vi "FTW-ProjectItemManager-ReadLinkedProjectItem.vi"(0 "Project Item Manager":refnum<class "FTW-ProjectItemManager.lvclass">, 5 "Linked Project Item Tag":string, 11 "error in":errorcluster) -> (4 "Project Item Manager out":refnum<class "FTW-ProjectItemManager.lvclass">, 6 "ProjectItem":refnum<vi>, 15 "error out":errorcluster)   [LabVIEW 2012, in "FTW-ProjectItemManager.lvclass"]
uses:
  FTW-ProjectItemManager.lvclass
  FTW-ProjectItemManager.lvclass/FTW-ProjectItemManager.ctl
panel:
  # "Inputs"
  # "Outputs"
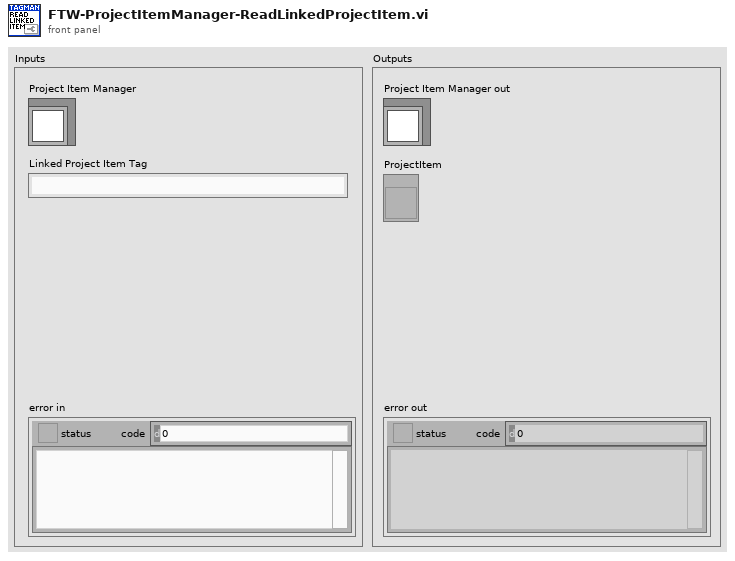
[diagram p1: front panel]
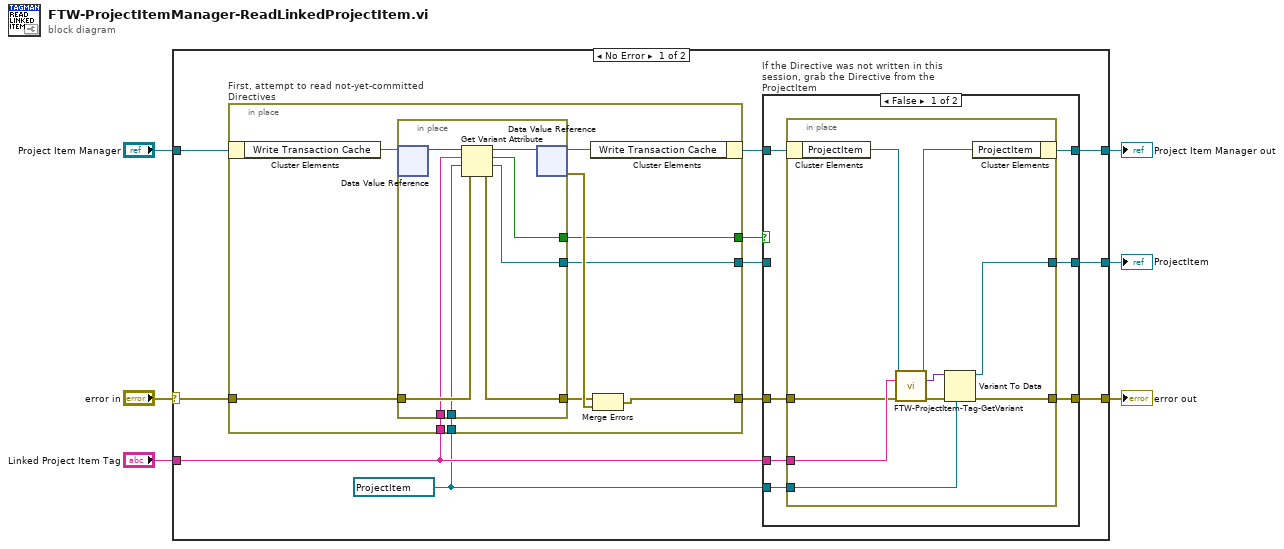
[diagram p0: block diagram]
diagram:
  n1 = case shown="No Error" "error in" {
    selector: "error in" -> [w13 w56]
    tunnel: [w7 w56] -> w6
    tunnel: [w17 w55] -> w4
    tunnel: "Project Item Manager" -> [w16 w55]
    tunnel: "Linked Project Item Tag" -> [w14 _]
    tunnel: [w8 _] -> w1
    frame No Error {
      w9 = refnum<vi> refnum ("Linked Project Item")
      n2 = in-place "First, attempt to read not-yet-committed Directives" {
        in-place-border: w13 -> [w46]
        in-place-border: [w39] -> w12
        in-place-border: w14 -> [w45]
        in-place-border: w9 -> [w44]
        in-place-border: [w38] -> w11
        in-place-border: [w37] -> w10
        n3 = in-place-cluster #1(w16) -> ("Write Transaction Cache"=w43:refnum<data-value>)
        n4 = in-place {
          in-place-border: w46 -> [w54]
          in-place-border: [w53] -> w40
          in-place-border: w45 -> [w52]
          in-place-border: w44 -> [w51]
          in-place-border: [w48] -> w38
          in-place-border: [w47] -> w37
          n5 = in-place-dvr #2(w43) -> (w50:variant)  [unwired: 1 out]
          n6 = Get Variant Attribute(Variant=w50, name=w52, default value (empty Variant)=w51, error in=w54) -> (duplicate Variant=w49:variant, found=w48:bool, value=w47:refnum<vi>, error out=w53:errorcluster)
          n7 = in-place-dvr #2(w49) -> (w42:refnum<data-value>, w41:errorcluster)
        }
        n8 = in-place-cluster #1("Write Transaction Cache"=w42) -> (w15:refnum<class "FTW-ProjectItemManager.lvclass">)
        n9 = Merge Errors(w40, w41) -> (w39:errorcluster)
      }
      n10 = case "If the Directive was not written in this\nsession, grab the Directive from the ProjectItem" shown="False" w11 {
        tunnel: [w23 w35] -> w8
        tunnel: [w18 w36] -> w17
        tunnel: [w22 w34] -> w7
        tunnel: w15 -> [w19 w36]
        tunnel: w9 -> [w24 _]
        tunnel: w14 -> [w21 _]
        tunnel: w12 -> [w20 w34]
        tunnel: w10 -> [_ w35]
        frame False {
          n11 = in-place {
            in-place-border: w24 -> [w33]
            in-place-border: [w32] -> w23
            in-place-border: [w31] -> w22
            in-place-border: w21 -> [w29]
            in-place-border: w20 -> [w28]
            n12 = in-place-cluster #3(w19) -> ("ProjectItem"=w26:refnum<vi>)
            n13 = call "FTW-ProjectItem-Tag-GetVariant.vi"("ProjectItem"=w26, "Tag Name"=w29, "error in"=w28) -> ("ProjectItem out"=w25:refnum<vi>, "Tag Value"=w30:variant, "error out"=w27:errorcluster)  [unwired: 8 in, 2 out]
            n14 = Variant To Data(error in=w27, type=w33, Variant=w30) -> (data=w32:refnum<vi>, error out=w31:errorcluster)
            n15 = in-place-cluster #3("ProjectItem"=w25) -> (w18:refnum<class "FTW-ProjectItemManager.lvclass">)
          }
        }
        frame True {
        }
      }
    }
    frame Error {
    }
  }
  "error out" <- w6
  "Project Item Manager out" <- w4
  "ProjectItem" <- w1
